vi "GlobalVI.vi"() -> ()   [LabVIEW 2019]
panel:
  in  "All UI Loop Stop":bool
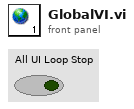
[diagram p1: front panel]
diagram:
